vi "TPNPT_MedianFilter.vi"(0 "Values":dbl[](array[numeric]) format="%.2f", 1 "last value":dbl format="%.2f", 2 "Number of samples":i32, 4 "index":i32, 5 "rank":i32=2) -> (7 "average":dbl format="%.2f", 8 "Values out":dbl[](array[numeric]) format="%.2f")   [LabVIEW 2016]
uses:
  <vilib>/Analysis/NI_AALBase.lvlib
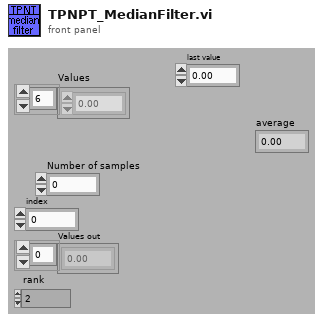
[diagram p1: front panel]
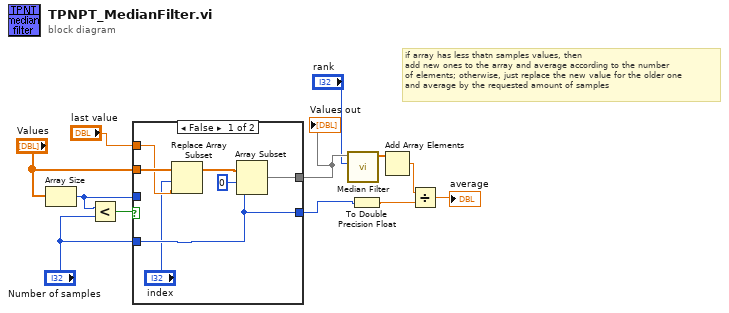
[diagram p0: block diagram]
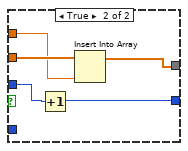
[diagram p2: hidden frame]
diagram:
  # "if array has less thatn samples values, then\nadd new ones to the array and average according to the number\nof elements; otherwise, just replace the new value for the older one\nand average by the requested amount of samples"
  n1 = Array Size(array="Values") -> (size(s)=w4:i32)
  n2 = Less?(x=w4, y="Number of samples") -> (x < y?=w6:bool)
  n3 = case shown="False" w6 {
    tunnel: [w18 w22] -> w3
    tunnel: "Values" -> [w16 w24]
    tunnel: [w17 w20] -> w8
    tunnel: "Number of samples" -> [w17 _]
    tunnel: "last value" -> [w14 w23]
    tunnel: w4 -> [_ w21]
    frame False {
      n4 = Replace Array Subset(array=w16, new element=w14, index="index") -> (w15:dbl[])
      n5 = Array Subset(array=w15, index=0 ("Array Index"), length=w17) -> (w18:dbl[])
    }
    frame True {
      n6 = Increment(x=w21) -> (x+1=w20:i32)
      n7 = Insert Into Array(array=w24, new element=w23) -> (w22:dbl[])  [unwired: 1 in]
    }
  }
  "Values out" <- w3
  n8 = call <vilib>:"Median Filter.vi"("left rank"="rank", "X"=w3) -> ("Filtered X"=w2:dbl[])  [unwired: 1 in, 8 out]
  n9 = To Double Precision Float(number=w8) -> (double precision float=w11:dbl)
  n10 = Add Array Elements(numeric array=w2) -> (sum=w12:dbl)
  n11 = Divide(x=w12, y=w11) -> (x/y=→"average":dbl)
